vi "Bairstow_s&r from P(x).vi"(8 "threshold":dbl=0.001, 9 "r in":dbl, 10 "s in":dbl, 11 "P(x)":dbl[](array[numeric])) -> (2 "r out":dbl, 3 "s out":dbl)   [LabVIEW 2020, in "NI_AALPro.lvlib"]
uses:
  <vilib>/Analysis/NI_AALPro.lvlib
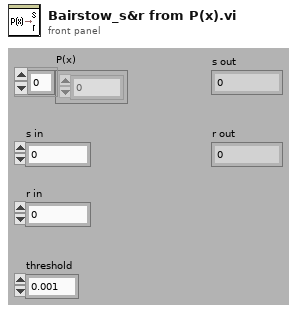
[diagram p1: front panel]
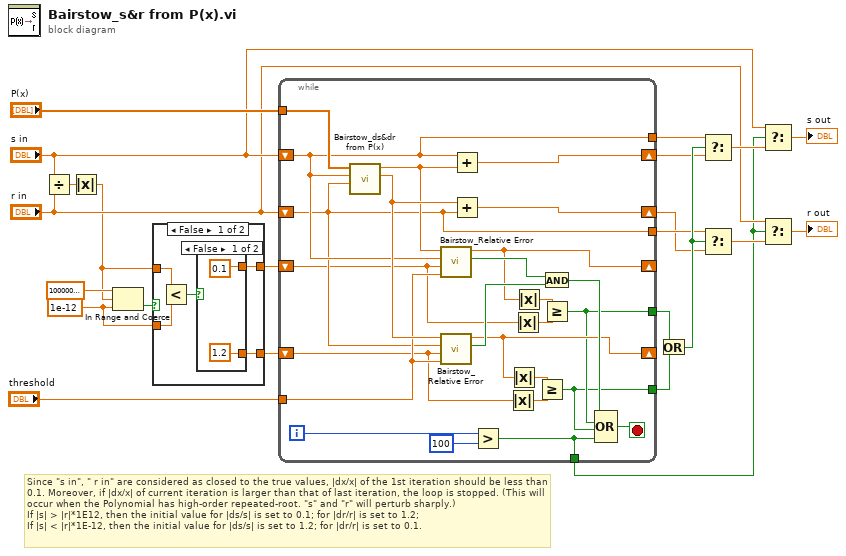
[diagram p0: block diagram]
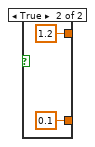
[diagram p2: hidden frame]
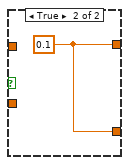
[diagram p3: hidden frame]
diagram:
  w9 = 1e-12 ("upper limit")
  # "Since \"s in\", \" r in\" are considered as closed to the true values, |dx/x| of the 1st iteration should be less than 0.1. Moreover, if |dx/x| of current iteration is larger than that of last iteration, the loop is stopped. (This will occur when the Polynomial has high-order repeated-root. \"s\" and \"r\" will perturb sharply.) \nIf |s| > |r|*1E12, then the initial value for |ds/s| is set to 0.1; for |dr/r| is set to 1.2;\nIf |s| < |r|*1E-12, then the initial value for |ds/s| is set to 1.2; for |dr/r| is set to 0.1."
  n1 = Divide(x="s in", y="r in") -> (x/y=w14:dbl)
  n2 = Absolute Value(x=w14) -> (abs(x)=w10:dbl)
  n3 = In Range and Coerce(upper limit=1000000000000.0, x=w10, lower limit=w9) -> (In Range?=w12:bool)  [unwired: 1 out]
  n4 = case shown="False" w12 {
    tunnel: [w25 w33] -> w22
    tunnel: [w24 w33] -> w11
    tunnel: w10 -> [w28 _]
    tunnel: w9 -> [w27 _]
    frame False {
      n5 = Less?(x=w28, y=w27) -> (x < y?=w26:bool)
      n6 = case shown="False" w26 {
        tunnel: [0.1 1.2] -> w25
        tunnel: [1.2 0.1] -> w24
        frame False {
        }
        frame True {
        }
      }
    }
    frame True {
      w33 = 0.1
    }
  }
  n7 = while {
    tunnel: "P(x)" -> [w58]
    shift-right: [w50] -> w4
    shift-left: "s in" -> [w47]
    shift-right: [w57] -> w2
    shift-left: "r in" -> [w46]
    shift-right: [w45] -> _
    shift-left: w22 -> [w43]
    shift-right: [w36] -> _
    shift-left: w11 -> [w39]
    tunnel: "threshold" -> [w53]
    tunnel: [w47] -> w5
    tunnel: [w46] -> w3
    tunnel: [w38] -> w1
    tunnel: [w35] -> w8
    tunnel: [w34] -> w7
    i -> [w52]
    stop <- w48 stop-if-true
    n8 = call <vilib>:"Bairstow_ds&dr from P(x).vi"("r"=w46, "s"=w47, "P(x)"=w58) -> ("dr"=w56:dbl, "ds"=w49:dbl)  [unwired: 7 in]
    n9 = call <vilib>:"Bairstow_Relative Error.vi"("threshold"=w53, "dx/x in"=w43, "x"=w47, "dx"=w49) -> ("less eps"=w55:bool, "dx/x out"=w45:dbl)  [unwired: 6 in]
    n10 = call <vilib>:"Bairstow_Relative Error.vi"("threshold"=w53, "dx/x in"=w39, "x"=w46, "dx"=w56) -> ("less eps"=w54:bool, "dx/x out"=w36:dbl)  [unwired: 6 in]
    n11 = Add(x=w47, y=w49) -> (x+y=w50:dbl)
    n12 = Add(x=w56, y=w46) -> (x+y=w57:dbl)
    n13 = Greater?(x=w52, y=100) -> (0:w38:bool)
    n14 = Absolute Value(x=w39) -> (abs(x)=w40:dbl)
    n15 = Absolute Value(x=w36) -> (abs(x)=w41:dbl)
    n16 = Absolute Value(x=w43) -> (abs(x)=w44:dbl)
    n17 = Absolute Value(x=w45) -> (abs(x)=w42:dbl)
    n18 = Greater Or Equal?(x=w41, y=w40) -> (x >= y?=w34:bool)
    n19 = And(x=w55, y=w54) -> (x .and. y?=w37:bool)
    n20 = Greater Or Equal?(x=w42, y=w44) -> (x >= y?=w35:bool)
    n21 = Compound Arithmetic op=OR(w37, w35, w34, w38) -> (w48:bool)
  }
  n22 = Or(x=w8, y=w7) -> (x .or. y?=w6:bool)
  n23 = Select(t=w5, s=w6, f=w4) -> (s? t:f=w20:dbl)
  n24 = Select(t=w3, s=w6, f=w2) -> (s? t:f=w19:dbl)
  n25 = Select(t="s in", s=w1, f=w20) -> (s? t:f=→"s out":dbl)
  n26 = Select(t="r in", s=w1, f=w19) -> (s? t:f=→"r out":dbl)
